vi "box.vi"(8 "error in (no error)":errorcluster, 10 "Plot 1 Data":dbl[](array[numeric])=[18.0, 19.0, 54.0, 83.0, 57.0, 45.0, 20.0, 0.0, 1.0, 54.0, -100.0, 120.0, -80.0]) -> (0 "error out":errorcluster, 1 "min":dbl, 2 "max":dbl, 3 "Box Plot":cluster{dbl[], dbl[]}[](graph)=[{[7.857142857142858, 2.142857142857143, 2.142857142857143, 7.857142857142858, 7.857142857142858, 2.142857142857143, 2.142857142857143], [20.0, 20.0, 0.75, 0.75, 54.75, 54.75, 20.0]}, {[], []}, {[5.0, 5.0, 5.0], [-100.0, 120.0, -80.0]}, {[5.0, 5.0], [54.75, 101.0]}, {[5.0, 5.0], [0.75, -61.0]}, {[6.428571428571429, 3.571428571428571], [101.0, 101.0]}, {[6.428571428571429, 3.571428571428571], [-61.0, -61.0]}, {[17.857142857142858, 12.142857142857142, 12.142857142857142, 17.857142857142858, 17.857142857142858, 12.142857142857142, 12.142857142857142], [8.5, 8.5, 1.5, 1.5, 38.5, 38.5, 8.5]}, {[], []}, {[15.0, 15.0], [100.0, -90.0]}, {[15.0, 15.0], [38.5, 64.0]}, {[15.0, 15.0], [1.5, -47.0]}, {[16.428571428571427, 13.571428571428571], [64.0, 64.0]}, {[16.428571428571427, 13.571428571428571], [-47.0, -47.0]}])   [LabVIEW 2022 SP3]
uses:
  LabVIEW Box Plots 2014/Box Plots Library/Box Plots.lvlib
panel:
  out "Value":cluster{dbl[], dbl[]}[](array[cluster])
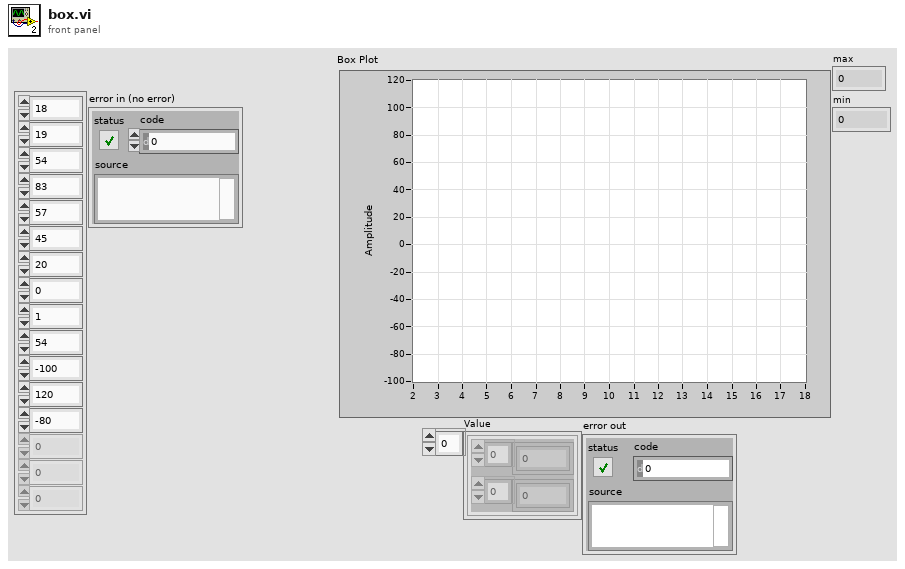
[diagram p1: front panel]
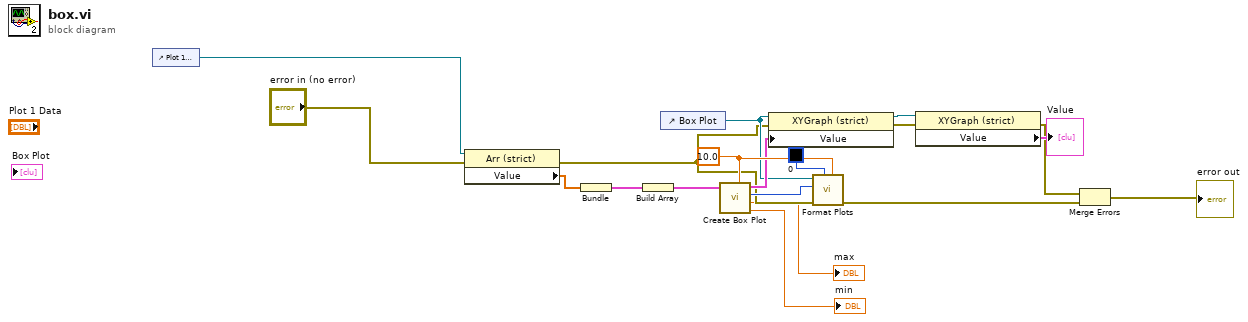
[diagram p0: block diagram]
diagram:
  w17 = 10.0 ("Width per Box Plot")
  n1 = control-ref of="Plot 1 Data"() -> (w3:refnum<vi>)
  n2 = property class="Arr (strict)"(reference=w3, error in="error in (no error)") -> (error out=w5:errorcluster, "Value"=w11:dbl[])  [unwired: 1 out]
  n3 = Bundle("Value"=w11) -> (w10:cluster{"Value":dbl[]})  [unwired: 1 in]
  n4 = Build Array(w10) -> (w18:cluster{"Value":dbl[]}[])
  n5 = control-ref of="Box Plot"() -> (w15:refnum<vi>)
  n6 = call "Create Box Plot.vi"("Width per Box Plot"=w17, "Raw Box Plot Data"=w18) -> ("min"=→"min":dbl, "max"=→"max":dbl, "Number of Plots"=w19:i32, "Box Plots"=w16:cluster{dbl[], dbl[]}[])  [unwired: 6 in]
  n7 = property class="XYGraph (strict)"(reference=w15, error in=w5, "Value"=w16) -> (reference out=w13:refnum<vi>, error out=w6:errorcluster)
  n8 = call "Format Plots.vi"("Box Plot Width"=w17, "Line Color"=u32 0, "error in (no error)"=w5, "Number of Plots"=w19, "XY Graph"=w15) -> ("error out"=w8:errorcluster)  [unwired: 6 in]
  n9 = property class="XYGraph (strict)"(reference=w13, error in=w6) -> (error out=w7:errorcluster, "Value"=→"Value":cluster{dbl[], dbl[]}[])  [unwired: 1 out]
  n10 = Merge Errors(w7, w8) -> (→"error out":errorcluster)
